vi "test Import Export GE Reflective Memory.vi"(8 "error in (no error)":errorcluster, 11 "TestCase in":refnum<class "Import Export Test.lvclass">) -> (0 "error out":errorcluster, 3 "TestCase out":refnum<class "Import Export Test.lvclass">)   [LabVIEW 2017, in "Import Export Test.lvclass"]
uses:
  Import Export Test.lvclass
  Import Export Test.lvclass/Import Export Test.ctl
  <vilib>/addons/_JKI Toolkits/VI Tester/TestCase.llb/TestCase.lvclass
  Scripting API/Data Sharing Framework Custom Device Scripting.lvlib
  niveristand-custom-device-testing-tools/VeriStandTestUtilities/VeriStandTestUtilities.lvlib
  C:/Program Files (x86)/National Instruments/LabVIEW 2017/vi.lib/addons/_JKI Toolkits/VI Tester/TestCase.llb/TestCase.lvclass
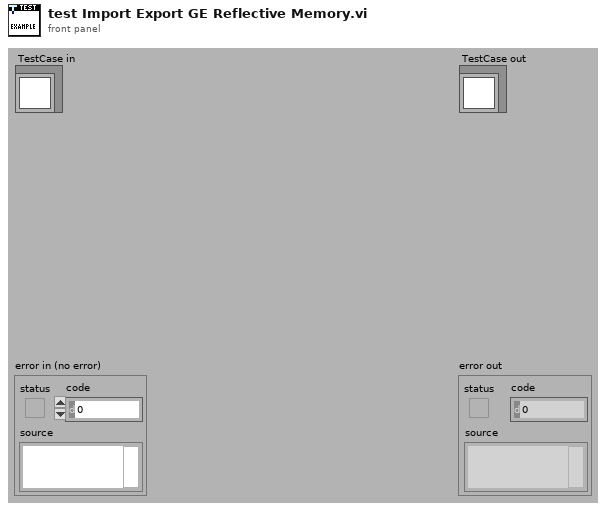
[diagram p1: front panel]
types:
  T1 = typedef "Custom Device API.lvlib/Custom Device Item Ref.ctl" = u64
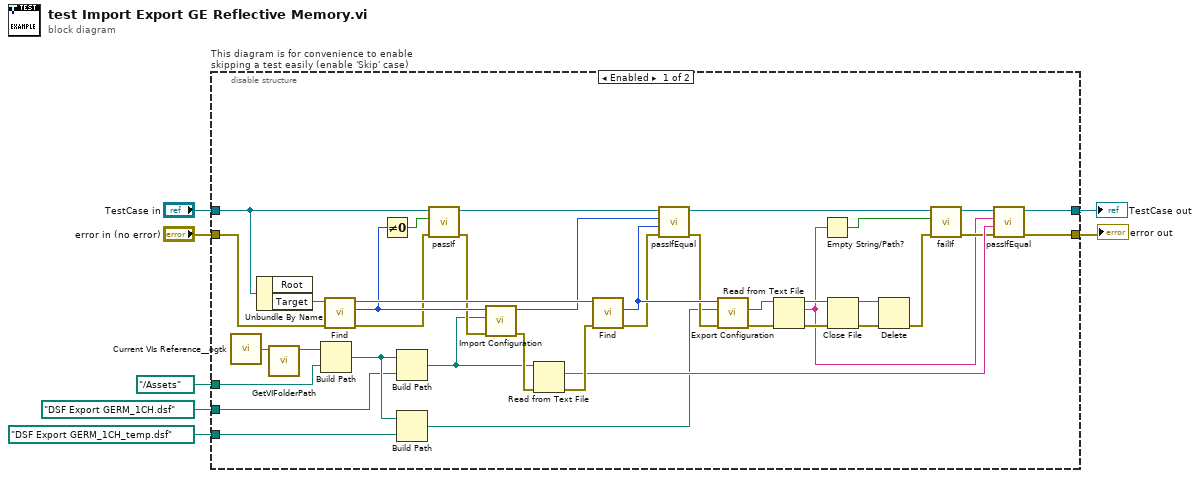
[diagram p0: block diagram]
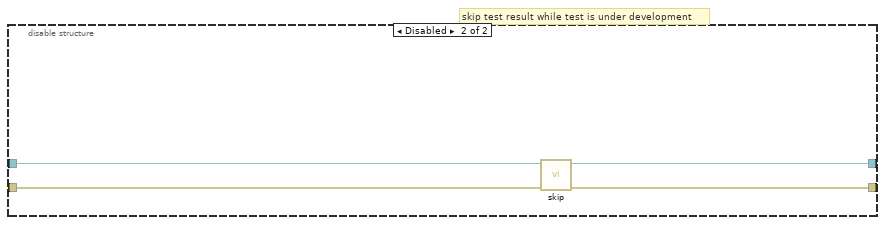
[diagram p2: hidden frame]
diagram:
  n1 = disable-structure "This diagram is for convenience to enable skipping a test easily (enable 'Skip' case)" shown="Enabled" {
    disable-tunnel: "TestCase in" -> [w37 w49]
    disable-tunnel: [w22 w47] -> w4
    disable-tunnel: [w21 w48] -> w6
    disable-tunnel: "error in (no error)" -> [w44 w46]
    disable-tunnel: path "DSF Export GERM_1CH_temp.dsf" ("VI Folder Path out") -> [w19 _]
    disable-tunnel: path "../Assets" ("VI Folder Path out") -> [w17 _]
    disable-tunnel: path "DSF Export GERM_1CH.dsf" ("VI Folder Path out") -> [w15 _]
    frame Enabled {
      n2 = call <userlib>:"Current VIs Reference__ogtk.vi"() -> ("Current VI's reference"=w43:refnum<vi>)  [unwired: 5 in]
      n3 = Unbundle By Name(w37) -> ("Target"=w45:refnum<k24>)  [unwired: 1 out]
      n4 = call "GetVIFolderPath.vi"("VI Reference in"=w43) -> ("VI Folder Path out"=w20:path)  [unwired: 9 in, 1 out]
      n5 = Build Path(base path=w20, name or relative path=w17) -> (appended path=w16:path)
      n6 = call "Find.vi"("error in"=w44, "target in"=w45) -> ("error out"=w26:errorcluster, "data sharing framework custom device"=w40:T1, "target out"=w42:refnum<k24>)  [unwired: 7 in]
      n7 = Not Equal To 0?(x=w40) -> (x != 0?=w31:bool)
      n8 = Build Path(base path=w16, name or relative path=w15) -> (appended path=w14:path)
      n9 = Build Path(base path=w16, name or relative path=w19) -> (appended path=w18:path)
      n10 = call-dynamic "passIf.vi"("error in (no error)"=w26, "pass"=w31, "TestCase in"=w37) -> ("error out"=w25:errorcluster, "TestCase out"=w41:refnum<class "Import Export Test.lvclass">)  [unwired: 7 in]
      n11 = call "Import Configuration.vi"("error in"=w25, "configuration file path"=w14, "data sharing framework custom device"=w40) -> ("error out"=w35:errorcluster, "data sharing framework custom device"=w39:T1)  [unwired: 7 in]
      n12 = Read from Text File(file (use dialog)=w14, error in=w35) -> (text=w29:string, error out=w34:errorcluster)  [unwired: 2 in, 2 out]
      n13 = call "Find.vi"("error in"=w34, "target in"=w42) -> ("error out"=w24:errorcluster, "data sharing framework custom device"=w38:T1)  [unwired: 7 in, 1 out]
      n14 = call-dynamic "passIfEqual.vi"("error in (no error)"=w24, "y"=w38, "x"=w39, "TestCase in"=w41) -> ("error out"=w23:errorcluster, "TestCase out"=w32:refnum<class "Import Export Test.lvclass">)  [unwired: 6 in]
      n15 = call "Export Configuration.vi"("error in"=w23, "configuration file path"=w18, "data sharing framework custom device"=w38) -> ("error out"=w33:errorcluster, "actual configuration file path"=w36:path)  [unwired: 6 in, 1 out]
      n16 = Read from Text File(file (use dialog)=w36, error in=w33) -> (refnum out=w13:refnum<file>, text=w8:string, error out=w12:errorcluster)  [unwired: 2 in, 1 out]
      n17 = Empty String/Path?(string/path=w8) -> (empty?=w30:bool)
      n18 = Close File(refnum=w13, error in=w12) -> (path=w11:path, error out=w10:errorcluster)
      n19 = Delete(path (use dialog)=w11, error in=w10) -> (error out=w9:errorcluster)  [unwired: 3 in, 2 out]
      n20 = call-dynamic "failIf.vi"("error in (no error)"=w9, "fail"=w30, "TestCase in"=w32) -> ("error out"=w27:errorcluster, "TestCase out"=w28:refnum<class "Import Export Test.lvclass">)  [unwired: 7 in]
      n21 = call-dynamic "passIfEqual.vi"("error in (no error)"=w27, "y"=w29, "x"=w8, "TestCase in"=w28) -> ("error out"=w21:errorcluster, "TestCase out"=w22:refnum<class "Import Export Test.lvclass">)  [unwired: 6 in]
    }
    frame Disabled {
      # "skip test result while test is under development"
      n22 = call <vilib>:"skip.vi"("error in (no error)"=w46, "TestCase in"=w49) -> ("error out"=w48:errorcluster, "TestCase out"=w47:refnum<class "Import Export Test.lvclass">)  [unwired: 8 in]
    }
  }
  "error out" <- w6
  "TestCase out" <- w4
